vi "DB Update Test Tree.vi"(8 "error in (no error)":errorcluster) -> (0 "error out":errorcluster)   [LabVIEW 2020]
uses:
  support/PCT FGV CMD.ctl
  support/REFs Name to ref convert.vi
  support/REF Single  Name to ref convert.vi
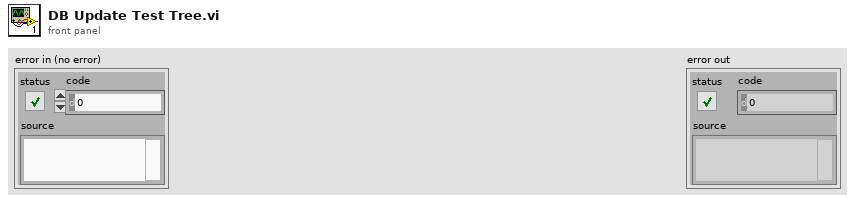
[diagram p1: front panel]
types:
  T1 = typedef "PCT FGV CMD.ctl" = enum16{"INIT", "GET", "SET"}
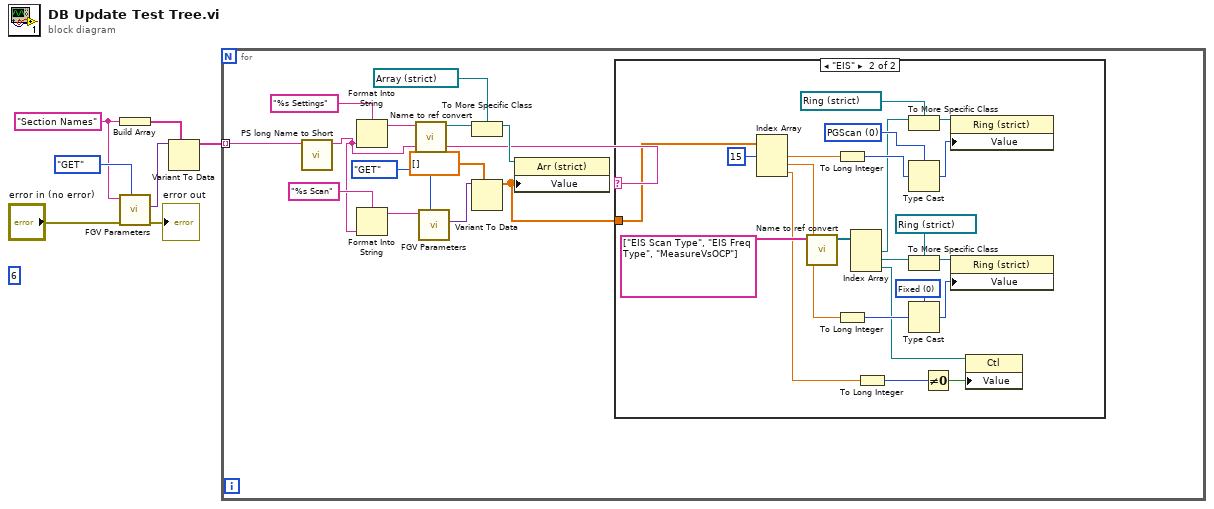
[diagram p0: block diagram]
diagram:
  w5 = "Section Names"
  (unwired) 6 ("index")
  n1 = Build Array(w5) -> (w4:string[])
  n2 = call "FGV Parameters.vi"("CMD"=PCT_FGV_CMD."GET", "error in (no error)"="error in (no error)", "Key"=w5) -> ("error out"=→"error out":errorcluster, "output"=w6:variant)  [unwired: 6 in, 1 out]
  n3 = Variant To Data(type=w4, Variant=w6) -> (data=w3:string[])  [unwired: 1 in, 1 out]
  n4 = for {
    tunnel: w3 -> [w11] mode=indexing
    n5 = call "PS long Name to Short.vi"("String"=w11) -> ("whole match"=w9:string)  [unwired: 10 in]
    n6 = Format Into String(format string="%s Settings", w9) -> (resulting string=w14:string)  [unwired: 2 in, 1 out]
    n7 = Format Into String(format string="%s Scan", w9) -> (resulting string=w17:string)  [unwired: 2 in, 1 out]
    n8 = call-poly "Name to ref convert.vi"("name"=w14) -> ("First REF"=w16:refnum<vi>)  [unwired: 10 in]
    n9 = call "FGV Parameters.vi"("CMD"=PCT_FGV_CMD."GET", "Key"=w17) -> ("output"=w19:variant)  [unwired: 7 in, 2 out]
    n10 = To More Specific Class(target class=refnum<vi> refnum ("CP Settings"), reference=w16) -> (specific class reference=w12:refnum<vi>)  [unwired: 1 in, 1 out]
    n11 = Variant To Data(type=dbl[] [] ("number"), Variant=w19) -> (data=w8:dbl[])  [unwired: 1 in, 1 out]
    n12 = property class="Arr (strict)"(reference=w12, "Value"=w8) -> ()  [unwired: 1 in, 2 out]
    n13 = case shown="\"EIS\"" w9 {
      tunnel: w8 -> [_ w42]
      frame "False", Default {
      }
      frame "EIS" {
        w30 = 0 items=["Fixed", "Scan"] ("EIS Freq Type")
        w36 = 0 items=["PGScan", "TimeScan", "Fixed"] ("EIS Scan Type")
        n14 = Index Array(array=w42, index #1=15 ("index")) -> (element #1=w35:dbl, element #2=w31:dbl, element #3=w27:dbl)  [unwired: 2 in]
        n15 = call-poly "Name to ref convert.vi"("Array in"=string[] ["EIS Scan Type", "EIS Freq Type", "MeasureVsOCP"] ("format string")) -> ("Array out"=w23:refnum<vi>[])  [unwired: 10 in]
        n16 = To Long Integer(number=w35) -> (32bit integer=w34:i32)
        n17 = To Long Integer(number=w31) -> (32bit integer=w32:i32)
        n18 = Index Array(array=w23) -> (element #1=w24:refnum<vi>, element #2=w22:refnum<vi>, element #3=w21:refnum<vi>)  [unwired: 3 in]
        n19 = To Long Integer(number=w27) -> (32bit integer=w26:i32)
        n20 = To More Specific Class(target class=refnum<vi> refnum ("EIS Scan Type"), reference=w24) -> (specific class reference=w37:refnum<vi>)  [unwired: 1 in, 1 out]
        n21 = Type Cast(type=w36, x=w34) -> (*(type *) &x=w33:i32)
        n22 = To More Specific Class(target class=refnum<vi> refnum ("EIS Freq Type"), reference=w22) -> (specific class reference=w29:refnum<vi>)  [unwired: 1 in, 1 out]
        n23 = Type Cast(type=w30, x=w32) -> (*(type *) &x=w28:i32)
        n24 = Not Equal To 0?(x=w26) -> (x != 0?=w25:bool)
        n25 = property class="Ring (strict)"(reference=w37, "Value"=w33) -> ()  [unwired: 1 in, 2 out]
        n26 = property class="Ring (strict)"(reference=w29, "Value"=w28) -> ()  [unwired: 1 in, 2 out]
        n27 = property class="Ctl"(reference=w21, "Value"=w25) -> ()  [unwired: 1 in, 2 out]
      }
    }
  }
